vi "API_Wait on Module Start.vi"(8 "error in (no error)":errorcluster, 10 "Wait for Event Sync?":bool) -> (0 "error out":errorcluster)   [LabVIEW 2015, in "Tool Module.lvlib"]
doc: "This is the API wrapper for the synchronize module events vi. This vi ensures the module and its caller have appropriately created and registered for events. This VI should be called after a module's caller registers for events, but before the module's caller's event structure starts."
uses:
  Tool Module.lvlib
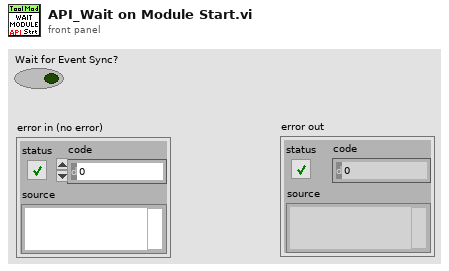
[diagram p1: front panel]
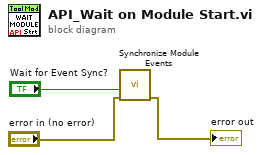
[diagram p0: block diagram]
diagram:
  n1 = call "Synchronize Module Events.vi"("error in (no error)"="error in (no error)", "Wait for Event Sync?"="Wait for Event Sync?") -> ("error out"=→"error out":errorcluster)  [unwired: 9 in]
